vi "PhotonTrackedTarget_CreateFromPacket.vi"(9 "StartByte":i32, 11 "RawData":u8[](array[numeric])) -> (1 "NextByte":i32, 3 "TrackedTarget":T1={"Yaw"=0.0, "Pitch"=0.0, "Area"=0.0, "Skew"=0.0, "TargetCorners"=[], "CameraToTarget"={"TRANSLATION"={"X"=0.0, "Y"=0.0}, "ROTATION"={"VALUE"=0.0, "COS"=1.0, "SIN"=0.0}, "xF"=FALSE}, "FiducialId"=0} {"CameraToTarget"."ROTATION"."SIN" format="%13.4f"; "CameraToTarget"."ROTATION"."COS" format="%13.4f"; "CameraToTarget"."ROTATION"."VALUE" format="%13.4f"; "CameraToTarget"."TRANSLATION"."Y" format="%14.3f"; "CameraToTarget"."TRANSLATION"."X" format="%14.3f"})   [LabVIEW 2020, in "PhotonVisionLib.lvlib"]
doc: "Internal function to parse the data for each target returned by PhotonCamera_GetLatestResult.\n\nInputs:\n - RawData -- Byte array containing the data to parse.\n\nOutputs:\n - TrackedTarget -- Parsed TrackedTarget cluster."
uses:
  PhotonVisionLib.lvlib
  TypeDef/PhotonTrackedTargetType.ctl
  TypeDef/TargetCornerType.ctl
  <vilib>/Rock Robotics/WPI/ThirdParty/JAS_Junk/TrajLib/TypeDef/TRANSFORM2D.ctl
  <vilib>/Rock Robotics/WPI/ThirdParty/JAS_Junk/TrajLib/TypeDef/TRANSLATION2D.ctl
  <vilib>/Rock Robotics/WPI/ThirdParty/JAS_Junk/TrajLib/TypeDef/ROTATION2D.ctl
  <vilib>/Rock Robotics/WPI/ThirdParty/JAS_Junk/TrajLib/Conv_Deg_Radians.vi
  <vilib>/Rock Robotics/WPI/ThirdParty/JAS_Junk/TrajLib/Rotation2d_CreateAngle.vi
  <vilib>/Rock Robotics/WPI/ThirdParty/JAS_Junk/TrajLib/Trajectory_Library.lvlib
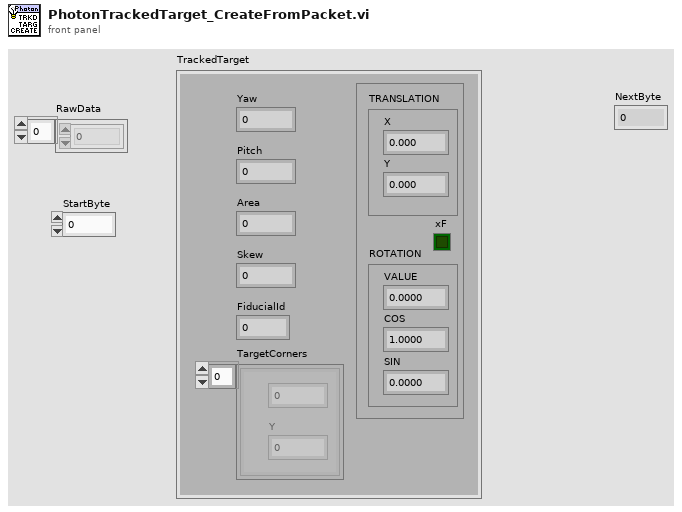
[diagram p1: front panel]
types:
  T1 = typedef "PhotonVisionLib.lvlib/PhotonTrackedTargetType.ctl" = cluster{"Yaw":dbl, "Pitch":dbl, "Area":dbl, "Skew":dbl, "TargetCorners":T2[], "CameraToTarget":T3, "FiducialId":i32}
  T2 = typedef "PhotonVisionLib.lvlib/TargetCornerType.ctl" = cluster{"X":dbl, "Y":dbl}
  T3 = typedef "Trajectory_Library.lvlib/TRANSFORM2D.ctl" = cluster{"TRANSLATION":T4, "ROTATION":T5, "xF":bool}
  T4 = typedef "Trajectory_Library.lvlib/TRANSLATION2D.ctl" = cluster{"X":dbl, "Y":dbl}
  T5 = typedef "Trajectory_Library.lvlib/ROTATION2D.ctl" = cluster{"VALUE":dbl, "COS":dbl, "SIN":dbl}
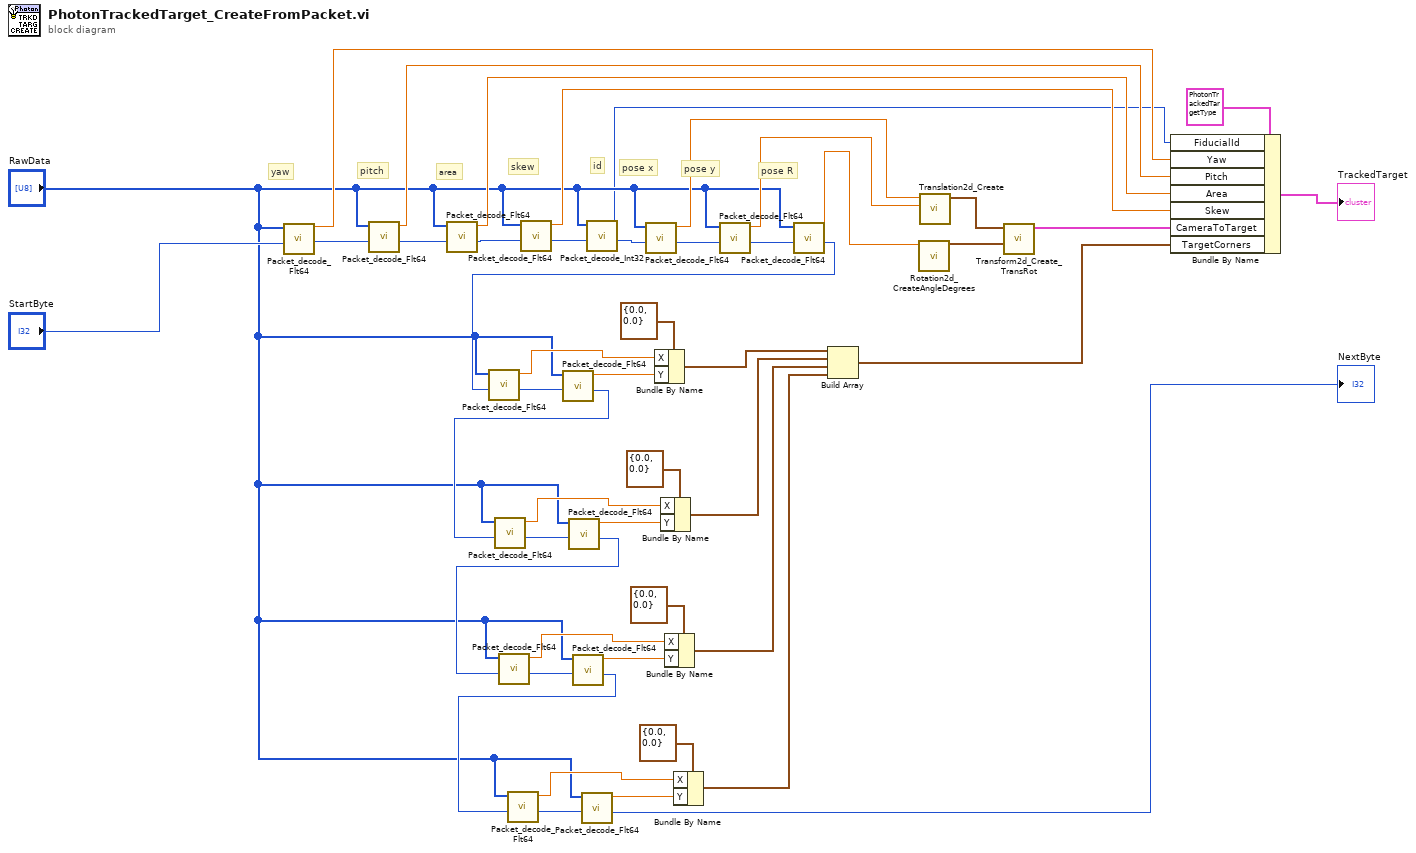
[diagram p0: block diagram]
diagram:
  # "id"
  # "pose R"
  # "pose y"
  # "pose x"
  # "skew"
  # "area"
  # "pitch"
  # "yaw"
  n1 = call "Packet_decode_Flt64.vi"("StartByte"="StartByte", "RawData"="RawData") -> ("NextByte"=w45:i32, "Flt64_Value"=w48:dbl)  [unwired: 8 in]
  n2 = call "Packet_decode_Flt64.vi"("StartByte"=w45, "RawData"="RawData") -> ("NextByte"=w43:i32, "Flt64_Value"=w44:dbl)  [unwired: 8 in]
  n3 = call "Packet_decode_Flt64.vi"("StartByte"=w43, "RawData"="RawData") -> ("NextByte"=w12:i32, "Flt64_Value"=w19:dbl)  [unwired: 8 in]
  n4 = call "Packet_decode_Flt64.vi"("StartByte"=w12, "RawData"="RawData") -> ("NextByte"=w4:i32, "Flt64_Value"=w11:dbl)  [unwired: 8 in]
  n5 = call "Packet_decode_Int32.vi"("StartByte"=w4, "RawData"="RawData") -> ("NextByte"=w3:i32, "Int32_Value"=w1:i32)  [unwired: 8 in]
  n6 = call "Packet_decode_Flt64.vi"("StartByte"=w3, "RawData"="RawData") -> ("NextByte"=w42:i32, "Flt64_Value"=w9:dbl)  [unwired: 8 in]
  n7 = call "Packet_decode_Flt64.vi"("StartByte"=w42, "RawData"="RawData") -> ("NextByte"=w41:i32, "Flt64_Value"=w8:dbl)  [unwired: 8 in]
  n8 = call "Packet_decode_Flt64.vi"("StartByte"=w41, "RawData"="RawData") -> ("NextByte"=w18:i32, "Flt64_Value"=w7:dbl)  [unwired: 8 in]
  n9 = call "Packet_decode_Flt64.vi"("StartByte"=w18, "RawData"="RawData") -> ("NextByte"=w40:i32, "Flt64_Value"=w37:dbl)  [unwired: 8 in]
  n10 = call "Packet_decode_Flt64.vi"("StartByte"=w40, "RawData"="RawData") -> ("NextByte"=w17:i32, "Flt64_Value"=w38:dbl)  [unwired: 8 in]
  n11 = call "Packet_decode_Flt64.vi"("StartByte"=w17, "RawData"="RawData") -> ("NextByte"=w36:i32, "Flt64_Value"=w33:dbl)  [unwired: 8 in]
  n12 = call "Packet_decode_Flt64.vi"("StartByte"=w36, "RawData"="RawData") -> ("NextByte"=w16:i32, "Flt64_Value"=w34:dbl)  [unwired: 8 in]
  n13 = call "Packet_decode_Flt64.vi"("StartByte"=w16, "RawData"="RawData") -> ("NextByte"=w32:i32, "Flt64_Value"=w29:dbl)  [unwired: 8 in]
  n14 = call "Packet_decode_Flt64.vi"("StartByte"=w32, "RawData"="RawData") -> ("NextByte"=w15:i32, "Flt64_Value"=w30:dbl)  [unwired: 8 in]
  n15 = call "Packet_decode_Flt64.vi"("StartByte"=w15, "RawData"="RawData") -> ("NextByte"=w28:i32, "Flt64_Value"=w25:dbl)  [unwired: 8 in]
  n16 = call "Packet_decode_Flt64.vi"("StartByte"=w28, "RawData"="RawData") -> ("NextByte"=→"NextByte":i32, "Flt64_Value"=w26:dbl)  [unwired: 8 in]
  n17 = Bundle By Name(cluster=T2 {"X"=0.0, "Y"=0.0} ("TargetCorner"), "X"=w37, "Y"=w38) -> (w24:T2)
  n18 = Bundle By Name(cluster=T2 {"X"=0.0, "Y"=0.0} ("TargetCorner"), "X"=w33, "Y"=w34) -> (w23:T2)
  n19 = Bundle By Name(cluster=T2 {"X"=0.0, "Y"=0.0} ("TargetCorner"), "X"=w29, "Y"=w30) -> (w22:T2)
  n20 = Bundle By Name(cluster=T2 {"X"=0.0, "Y"=0.0} ("TargetCorner"), "X"=w25, "Y"=w26) -> (w21:T2)
  n21 = Build Array(w24, w23, w22, w21) -> (w20:T2[])
  n22 = call <vilib>:"Rotation2d_CreateAngleDegrees.vi"("Angle_Degrees"=w7) -> ("ROTATION"=w6:T5)  [unwired: 10 in]
  n23 = call <vilib>:"Translation2d_Create.vi"("Y"=w8, "X"=w9) -> ("TRANSLATION"=w5:T4)  [unwired: 9 in]
  n24 = call <vilib>:"Transform2d_Create_TransRot.vi"("ROTATION"=w6, "TRANSLATION"=w5) -> ("TRANSFORM"=w10:T3)  [unwired: 9 in]
  n25 = Bundle By Name(cluster=T1 {"Yaw"=0.0, "Pitch"=0.0, "Area"=0.0, "Skew"=0.0, "TargetCorners"=[], "CameraToTarget"={"TRANSLATION"={"X"=0.0, "Y"=0.0}, "ROTATION"={"VALUE"=0.0, "COS"=1.0, "SIN"=0.0}, "xF"=FALSE}, "FiducialId"=0} ("PhotonTrackedTarget"), "FiducialId"=w1, "Yaw"=w48, "Pitch"=w44, "Area"=w19, "Skew"=w11, "CameraToTarget"=w10, "TargetCorners"=w20) -> (→"TrackedTarget":T1)
